vi "Bodies_Init_GVec.vi"(6 "Gravity Direction":dbl[](array[numeric]), 8 "error in (no error)":errorcluster, 9 "Negative Direction (T)":bool=TRUE, 10 "Gravity Axis (z)":T1=enum."Z", 11 "Bodies in":refnum<class "Bodies.lvclass">) -> (0 "error out":errorcluster, 3 "Bodies out":refnum<class "Bodies.lvclass">)   [LabVIEW 2015, in "Bodies.lvclass"]
uses:
  Bodies.lvclass
  xyzO.ctl
  Bodies.lvclass/Bodies.ctl
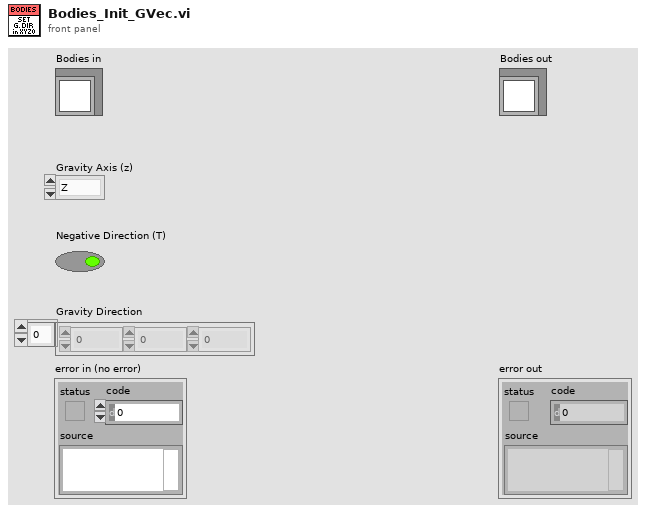
[diagram p1: front panel]
types:
  T1 = typedef "Bodies.lvclass/xyzO.ctl" = enum16{"X", "Y", "Z", "O"}
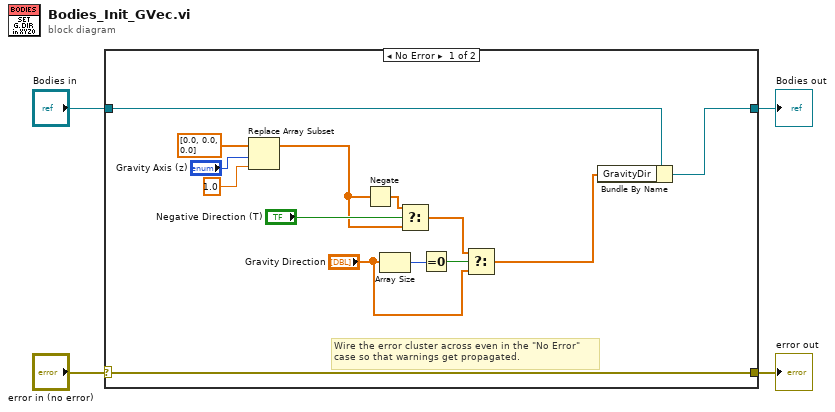
[diagram p0: block diagram]
diagram:
  n1 = case shown="No Error" "error in (no error)" {
    selector: "error in (no error)" -> [w18 w20]
    tunnel: [w18 w20] -> w3
    tunnel: [w16 w19] -> w1
    tunnel: "Bodies in" -> [w17 w19]
    frame No Error {
      # "Wire the error cluster across even in the \"No Error\"\ncase so that warnings get propagated."
      n2 = Replace Array Subset(array=dbl[] [0.0, 0.0, 0.0], new element=1.0 ("new element/subarray"), index="Gravity Axis (z)") -> (w7:dbl[])
      n3 = Negate(x=w7) -> (-x=w8:dbl[])
      n4 = Array Size(array="Gravity Direction") -> (size(s)=w15:i32)
      n5 = Select(t=w8, s="Negative Direction (T)", f=w7) -> (s? t:f=w6:dbl[])
      n6 = Equal To 0?(x=w15) -> (x = 0?=w14:bool)
      n7 = Select(t=w6, s=w14, f="Gravity Direction") -> (s? t:f=w5:dbl[])
      n8 = Bundle By Name(cluster=w17, "GravityDir"=w5) -> (w16:refnum<class "Bodies.lvclass">)
    }
    frame Error {
    }
  }
  "error out" <- w3
  "Bodies out" <- w1
